vi "go_to_wavelength.vi"(0 "Set Laser Position":dbl, 2 "Unit":u16(ring) items=["nm", "cm-1"], 11 "error in (no error)":errorcluster) -> (4 "Current Laser Position":dbl, 15 "error out":errorcluster)   [LabVIEW 2023]
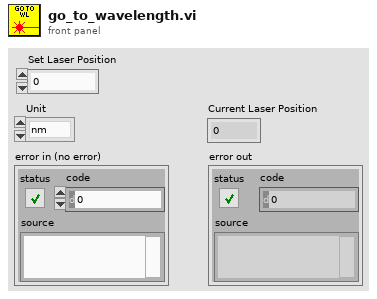
[diagram p1: front panel]
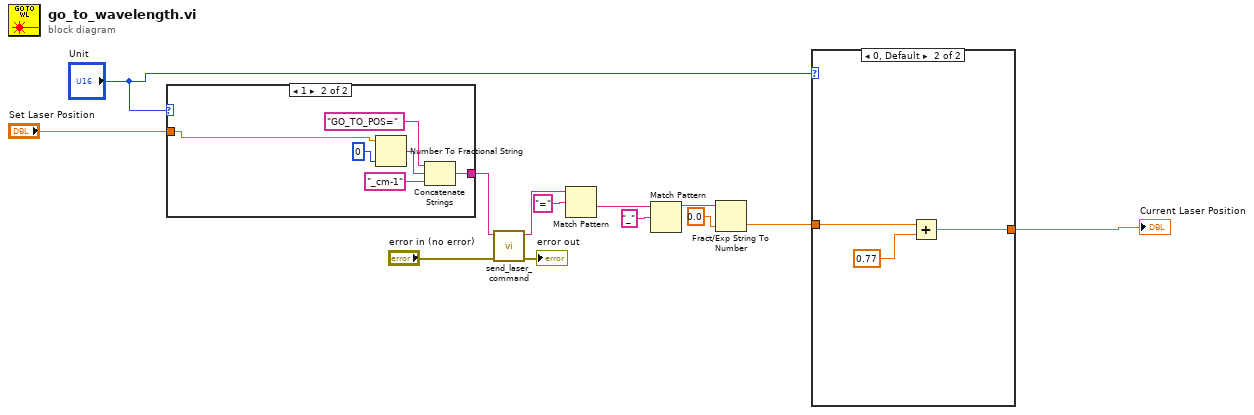
[diagram p0: block diagram]
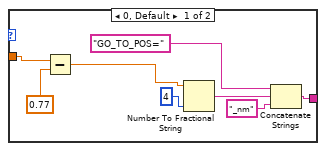
[diagram p3: hidden frame]
diagram:
  n1 = case shown="1" "Unit" {
    tunnel: [w17 w23] -> w13
    tunnel: "Set Laser Position" -> [w16 w22]
    frame 0, Default {
      n2 = Subtract(x=w16, y=0.77) -> (x-y=w15:dbl)
      n3 = Number To Fractional String(number=w15, precision (6)=i16 4) -> (F-format string=w19:string)  [unwired: 2 in]
      n4 = Concatenate Strings("GO_TO_POS=", w19, "_nm" ("string")) -> (w17:string)
    }
    frame 1 {
      n5 = Number To Fractional String(number=w22, precision (6)=i16 0) -> (F-format string=w25:string)  [unwired: 2 in]
      n6 = Concatenate Strings("GO_TO_POS=", w25, "_cm-1" ("string")) -> (w23:string)
    }
  }
  n7 = call "send_laser_command.vi"("error in (no error)"="error in (no error)", "String"=w13) -> ("error out"=→"error out":errorcluster, "data out"=w5:string)  [unwired: 8 in]
  n8 = Match Pattern(string=w5, regular expression="=") -> (after substring=w9:string)  [unwired: 1 in, 3 out]
  n9 = Match Pattern(string=w9, regular expression="_") -> (before substring=w7:string)  [unwired: 1 in, 3 out]
  n10 = Fract/Exp String To Number(string=w7, default (0 dbl)=0.0 ("number")) -> (number=w2:dbl)  [unwired: 2 in, 1 out]
  n11 = case shown="0, Default" "Unit" {
    tunnel: w2 -> [w28 w31]
    tunnel: [w28 w29] -> w1
    frame 1 {
    }
    frame 0, Default {
      n12 = Add(x=w31, y=0.77) -> (x+y=w29:dbl)
    }
  }
  "Current Laser Position" <- w1
